vi "Test Process Set Self as Error Handler.vi"(8 "error in (no error)":errorcluster, 11 "Process Test In":refnum<class "Process Test.lvclass">) -> (0 "error out":errorcluster, 3 "Process Test Out":refnum<class "Process Test.lvclass">)   [LabVIEW 2020, in "Process Test.lvclass"]
uses:
  Process Test.lvclass
  Framework/Process/Process.lvclass
  C:/Users/anton/Documents/GitHub/Triarc-Framework/source/Framework/Error Handler Interface/Error Handler Interface.lvclass
  Framework/Process/Process.lvclass/Process.ctl
  Framework/Process/Protected/Messaging/Enqueue Message.vi
  Framework/Process/Public/Lifecycle/Get Lifecycle State.vi
  <vilib>/Utility/error.llb/Clear Errors.vi
  <vilib>/Asteme/LUnit/Test Case.lvclass
  C:/Users/anton/Documents/GitHub/Triarc-Framework/source/Framework/Base/Base.lvclass
  C:/Users/anton/Documents/GitHub/Triarc-Framework/source/Framework/Process/Process.lvclass
  C:/Users/anton/Documents/GitHub/Triarc-Framework/source/Framework/Logging/Logging.lvclass
  C:/Users/anton/Documents/GitHub/Triarc-Framework/source/Framework Test/Base Class Test/Base Test.lvclass
  C:/Program Files (x86)/National Instruments/LabVIEW 2020/vi.lib/Asteme/LUnit/Test Case.lvclass
  C:/Users/anton/Documents/GitHub/Triarc-Framework/source/Framework Test/Process Test/Process Test.lvclass
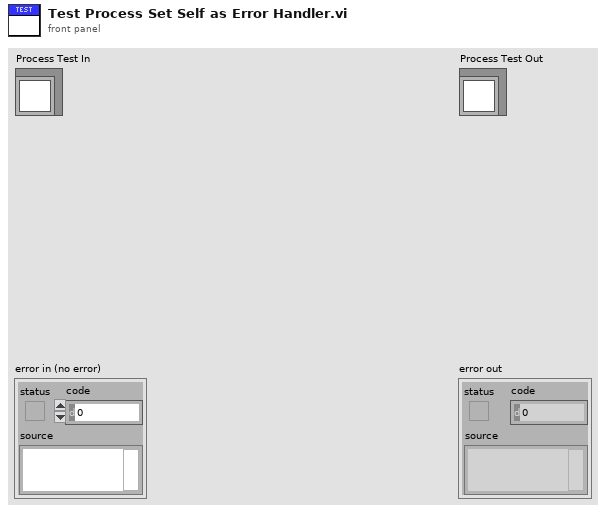
[diagram p1: front panel]
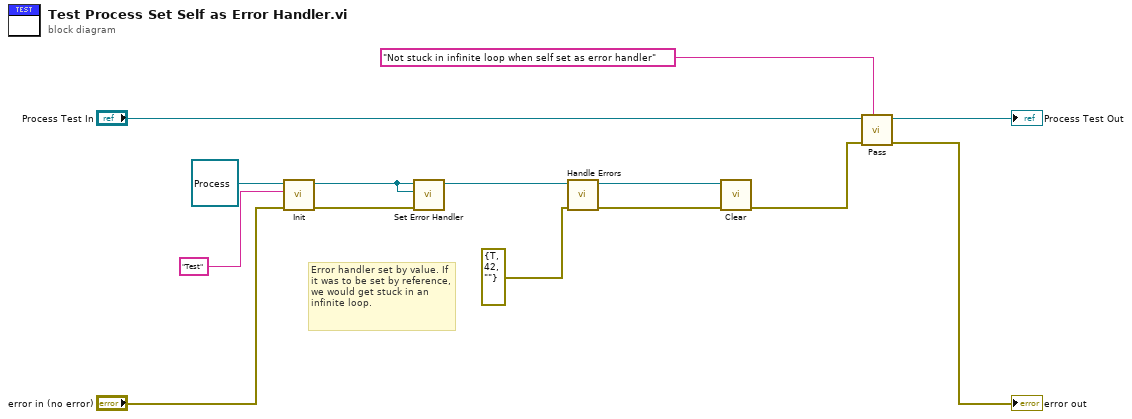
[diagram p0: block diagram]
diagram:
  # "Error handler set by value. If it was to be set by reference, we would get stuck in an infinite loop."
  n1 = call-dynamic "Init.vi"("error in (no error)"="error in (no error)", "Name"="Test", "Process In"=refnum<class "Process.lvclass"> refnum ("Process.lvclass")) -> ("error out"=w14:errorcluster, "Process Out"=w10:refnum<class "Process.lvclass">)  [unwired: 7 in]
  n2 = call "Set Error Handler.vi"("error in (no error)"=w14, "Error Handler"=w10, "Process In"=w10) -> ("Process Out"=w13:refnum<class "Process.lvclass">)  [unwired: 7 in, 1 out]
  n3 = call-dynamic "Handle Errors.vi"("error in (no error)"=errorcluster {"status"=TRUE, "code"=42, "source"=""} ("Mock Error"), "Process In"=w13) -> ("error out"=w9:errorcluster, "Process Out"=w8:refnum<class "Process.lvclass">)  [unwired: 8 in]
  n4 = call-dynamic "Clear.vi"("error in (no error)"=w9, "Process In"=w8) -> ("error out"=w7:errorcluster)  [unwired: 9 in]
  n5 = call <vilib>:"Pass.vi"("Description"="Not stuck in infinite loop when self set as error handler", "error in (no error)"=w7, "Test Case In"="Process Test In") -> ("error out"=→"error out":errorcluster, "Test Case Out"=→"Process Test Out":refnum<class "Process Test.lvclass">)  [unwired: 7 in]
